vi "CreateShiftRegisters.vi"(6 "error in":errorcluster, 9 "Loop in":refnum<class "Loop.lvclass">) -> (0 "error out":errorcluster, 3 "Loop out":refnum<class "Loop.lvclass">, 4 "createSR":string)   [LabVIEW 2014, in "Raspberry Pi Compatible Compiler for LabVIEW.lvlib" / "Loop.lvclass"]
uses:
  Loop.lvclass
  Loop.lvclass/Loop.ctl
  Python/Parsing/ClassTypeTD.ctl
  Python/Parsing/ListTypesTD.ctl
  ShiftRegister/ShiftRegister.lvclass/ShiftRegister.ctl
  Tunnel/Tunnel.lvclass/Tunnel.ctl
  RightShiftRegister/RightShiftRegister.lvclass
  Python/Parsing/Python Functions.lvlib
  Terminal/Terminal.lvclass
  Tunnel/Tunnel.lvclass
  ShiftRegister/ShiftRegister.lvclass
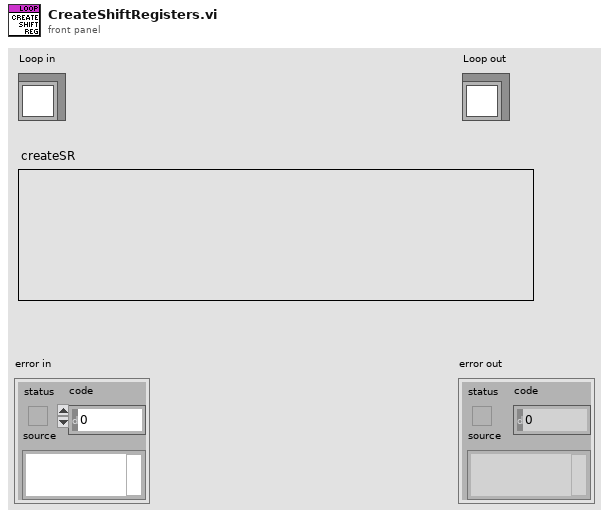
[diagram p1: front panel]
types:
  T1 = typedef "Raspberry Pi Compatible Compiler for LabVIEW.lvlib/Python Functions.lvlib/ListTypesTD.ctl" = enum16{"list", "tuple", "parameter list", "output list", "return values"}
  T2 = typedef "Raspberry Pi Compatible Compiler for LabVIEW.lvlib/Python Functions.lvlib/ClassTypeTD.ctl" = enum16{"class", "function"}
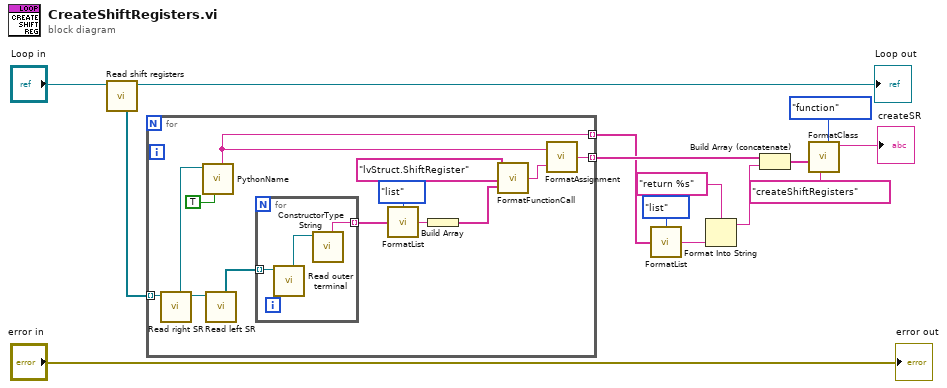
[diagram p0: block diagram]
diagram:
  n1 = call "Read shift registers.vi"("Loop in"="Loop in") -> ("Loop out"=→"Loop out":refnum<class "Loop.lvclass">, "shift registers"=w1:refnum<class "ShiftRegister.lvclass">[])  [unwired: 7 in]
  n2 = for {
    tunnel: w1 -> [w22] mode=indexing
    tunnel: [w25] -> w11 mode=indexing
    tunnel: [w23] -> w9 mode=indexing
    n3 = call "Read right SR.vi"("ShiftRegister in"=w22) -> ("ShiftRegister out"=w21:refnum<class "ShiftRegister.lvclass">, "right SR"=w20:refnum<class "RightShiftRegister.lvclass">)  [unwired: 7 in]
    n4 = call-dynamic "PythonName.vi"("add self"=TRUE, "GObject in"=w20) -> ("name"=w23:string)  [unwired: 6 in, 3 out]
    n5 = call "Read left SR.vi"("ShiftRegister in"=w21) -> ("left SR"=w19:refnum<class "LeftShiftRegister.lvclass">[])  [unwired: 7 in, 1 out]
    n6 = for {
      tunnel: w19 -> [w29] mode=indexing
      tunnel: [w28] -> w18 mode=indexing
      n7 = call "Read outer terminal.vi"("Tunnel in"=w29) -> ("outer terminal"=w30:refnum<class "Terminal.lvclass">)  [unwired: 7 in, 1 out]
      n8 = call "ConstructorTypeString.vi"("Terminal in"=w30) -> ("constructor string"=w28:string)  [unwired: 6 in, 2 out]
    }
    n9 = call "FormatList.vi"("values"=w18, "type"=ListTypesTD."list") -> ("python object"=w16:string)
    n10 = Build Array(w16) -> (w15:string[])
    n11 = call "FormatFunctionCall.vi"("parameters"=w15, "function"="lvStruct.ShiftRegister" ("format string")) -> ("python object"=w24:string)
    n12 = call "FormatAssignment.vi"("value"=w24, "name"=w23) -> ("python assignment"=w25:string)
  }
  n13 = call "FormatList.vi"("values"=w9, "type"=ListTypesTD."list") -> ("python object"=w7:string)
  n14 = Format Into String(format string="return %s", w7) -> (resulting string=w4:string)  [unwired: 2 in, 1 out]
  n15 = Build Array (concatenate)(w11, w4) -> (w5:string[])
  n16 = call "FormatClass.vi"("type"=ClassTypeTD."function", "name"="createShiftRegisters", "body"=w5) -> ("python"=→"createSR":string)  [unwired: 8 in]
  "error out" <- "error in"
